vi "Exemple d'utilisation simple - Capteur.vi"() -> ()   [LabVIEW 2013]
panel:
  out "Pressure":cluster{"Y":dbl[], "Y":dbl[]}[](graph)
  in  "Length":i32=250 caption="Length (ms)"
  in  "Online":bool
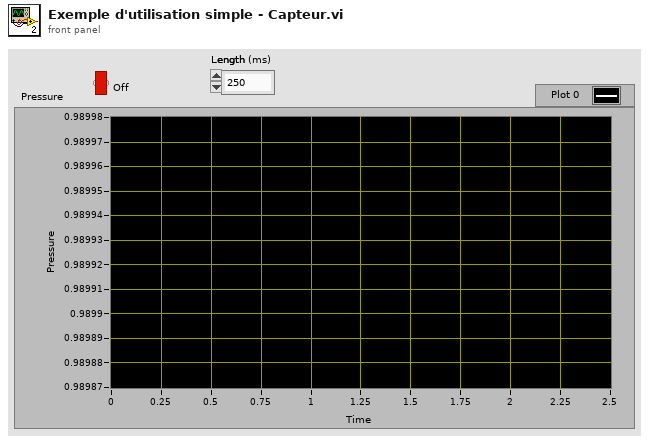
[diagram p1: front panel]
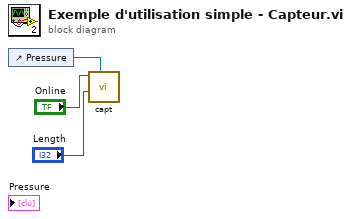
[diagram p0: block diagram]
diagram:
  n1 = control-ref of="Pressure"() -> (w2:refnum<vi>)
  n2 = call "capt.vi"("XY Graph Ref In"=w2, "Length"="Length", "Online"="Online") -> ()  [unwired: 8 in, 1 out]
